vi "MagicPin State.vi"(11 "error in":errorcluster) -> (8 "State":bool, 15 "error out":errorcluster)   [LabVIEW 2010]
uses:
  <vilib>/DAQmx/read.llb/DAQmx Read (Digital Bool 1Line 1Point).vi
  <vilib>/DAQmx/create/channels.llb/DAQmx Create Channel (DI-Digital Input).vi
  <vilib>/daqmx/miscellaneous.llb/DAQmx Fill In Error Info.vi
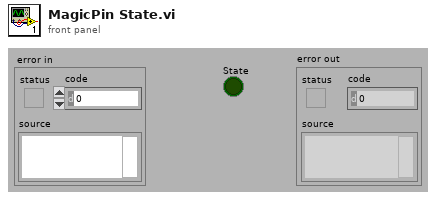
[diagram p1: front panel]
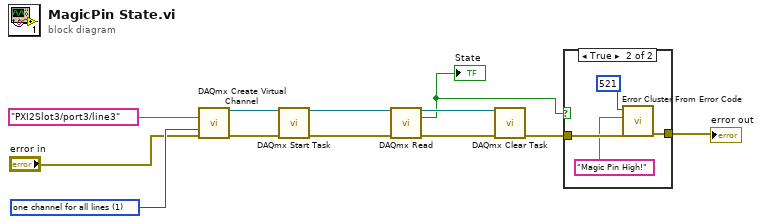
[diagram p0: block diagram]
diagram:
  w10 = 1 items=["one channel for each line", "one channel for all lines"] ("line grouping")
  n1 = call-poly <vilib>:"DAQmx Create Virtual Channel.vi"("lines"=tag "PXI2Slot3/port3/line3" ("Lines"), "line grouping"=w10, "error in"="error in") -> ("task out"=w12:refnum<k21>, "error out"=w11:errorcluster)  [unwired: 11 in]
  n2 = call <vilib>:"DAQmx Start Task.vi"("task/channels in"=w12, "error in"=w11) -> ("task out"=w9:refnum<k21>, "error out"=w8:errorcluster)  [unwired: 12 in]
  n3 = call-poly <vilib>:"DAQmx Read.vi"("task/channels in"=w9, "error in"=w8) -> ("task out"=w7:refnum<k21>, "data"=w2:bool, "error out"=w6:errorcluster)  [unwired: 11 in]
  "State" <- w2
  n4 = call <vilib>:"DAQmx Clear Task.vi"("task in"=w7, "error in"=w6) -> ("error out"=w3:errorcluster)  [unwired: 13 in]
  n5 = case shown="True" w2 {
    tunnel: w3 -> [w13 w17]
    tunnel: [w13 w16] -> w1
    frame False {
    }
    frame True {
      n6 = call <vilib>:"Error Cluster From Error Code.vi"("error in (no error)"=w17, "error message (\"\")"="Magic Pin High!" ("error message (\"\")"), "error code (0)"=521) -> ("error out"=w16:errorcluster)  [unwired: 6 in]
    }
  }
  "error out" <- w1
